vi "Power Supply.vi"() -> ()   [LabVIEW 2020]
uses:
  lv_waveforms_toolkit/lv_waveforms_toolkit.lvlib
panel:
  in  "Voltage":dbl(slide)=3.3 scale=0.0..5.0
  out "Error Out":errorcluster
  in  "stop":bool
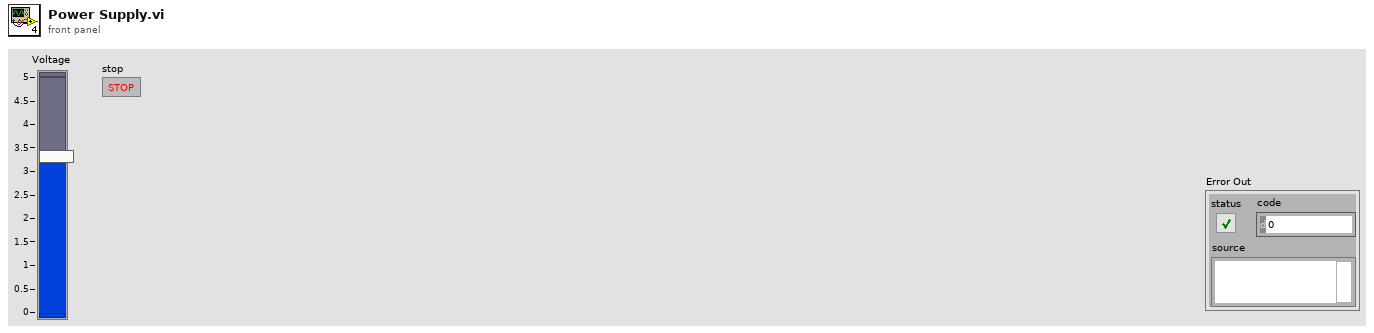
[diagram p1: front panel]
types:
  T1 = typedef "lv_waveforms_toolkit.lvlib/WFT Session.ctl" = cluster{"phdwf":i32, "Analog IO Configured":bool}
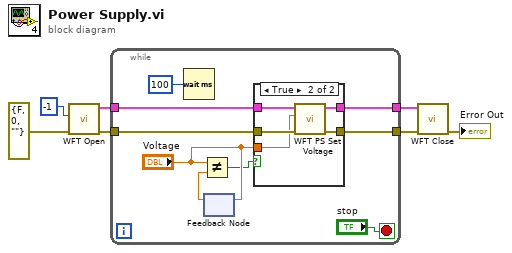
[diagram p0: block diagram]
diagram:
  n1 = call "WFT Open.vi"("Error In"=errorcluster {"status"=FALSE, "code"=0, "source"=""}, "idxDevice"=-1) -> ("Error Out"=w2:errorcluster, "WaveForms Session Out"=w1:T1)  [unwired: 7 in, 1 out]
  n2 = while {
    tunnel: [w11] -> w7
    tunnel: [w12] -> w6
    tunnel: w2 -> [w14]
    tunnel: w1 -> [w13]
    stop <- "stop" stop-if-true
    n3 = Wait (ms)(milliseconds to wait=u32 100) -> ()  [unwired: 1 out]
    n4 = feedback-in #1("Voltage") -> ()
    n5 = feedback #1() -> (w9:dbl)  [unwired: 1 in]
    n6 = Not Equal?(x="Voltage", y=w9) -> (x != y?=w8:bool)
    n7 = case shown="True" w8 {
      tunnel: w14 -> [w17 w23]
      tunnel: w13 -> [w18 w22]
      tunnel: [w17 w21] -> w12
      tunnel: [w18 w20] -> w11
      tunnel: "Voltage" -> [_ w19]
      frame False {
      }
      frame True {
        n8 = call "WFT PS Set Voltage.vi"("Error In"=w23, "Voltage"=w19, "WaveForms Session In"=w22) -> ("Error Out"=w21:errorcluster, "WaveForms Session Out"=w20:T1)  [unwired: 7 in]
      }
    }
  }
  n9 = call "WFT Close.vi"("Error In"=w6, "WaveForms Session In"=w7) -> ("Error Out"=→"Error Out":errorcluster)  [unwired: 8 in, 1 out]
